vi "Adv_GetControlCurrentCapabilities_native.vi"(6 "LightField Setting":string, 8 "error in (no error)":errorcluster, 9 "Enum Class":refnum<k24>, 10 "Control":refnum<vi>, 11 "LightField Automation in":refnum<class "LightField Automation.lvclass">) -> (0 "error out":errorcluster, 3 "LightField Automation out":refnum<class "LightField Automation.lvclass">)   [LabVIEW 2015, in "LightField Automation.lvclass"]
uses:
  LightField Automation.lvclass
  C:/Program Files/Princeton Instruments/LightField/AddInViews/PrincetonInstruments.LightFieldViewV3.dll
  Program Files/Princeton Instruments/LightField/AddInViews/PrincetonInstruments.LightFieldViewV3.dll
  <vilib>/Utility/error.llb/DialogType.ctl
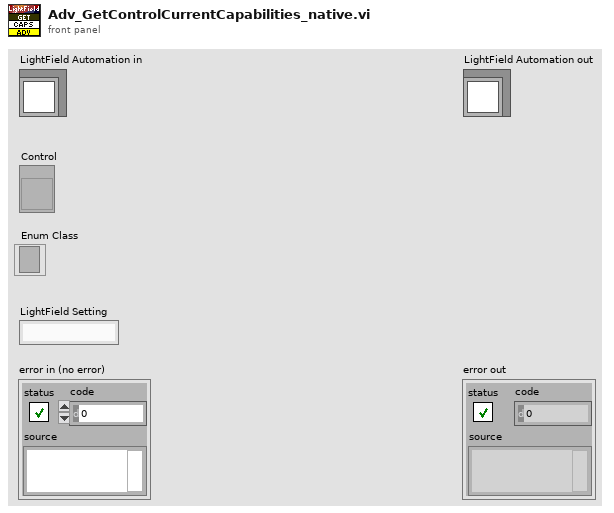
[diagram p1: front panel]
types:
  T1 = typedef "DialogType.ctl" = u16
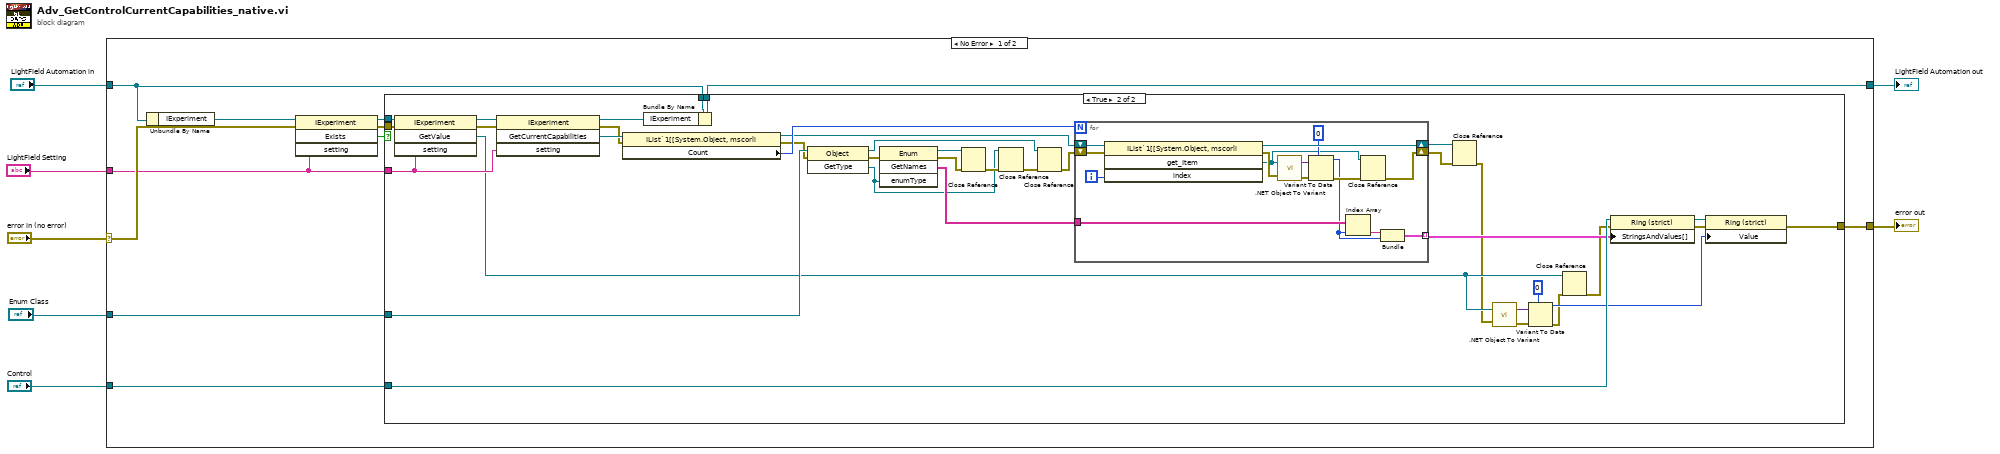
[diagram p0: block diagram]
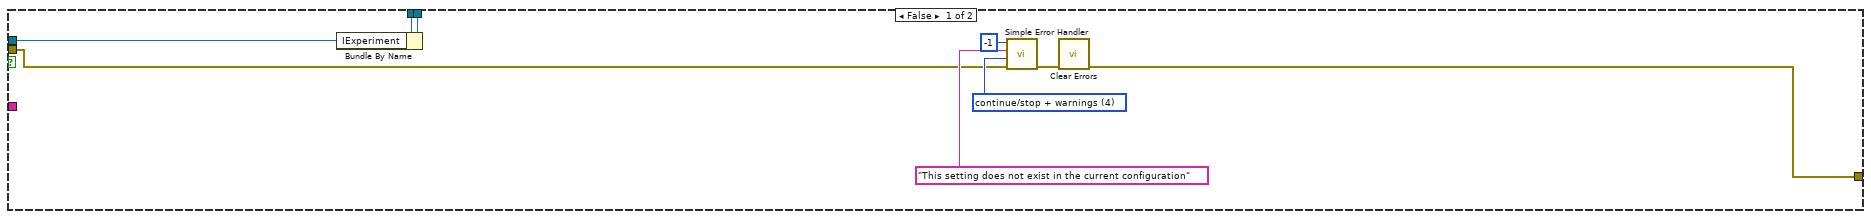
[diagram p2: hidden frame]
diagram:
  n1 = case shown="No Error" "error in (no error)" {
    selector: "error in (no error)" -> [w10 w82]
    tunnel: [w15 w82] -> w6
    tunnel: [w17 w81] -> w4
    tunnel: "LightField Automation in" -> [w18 w81]
    tunnel: "Control" -> [w16 _]
    tunnel: "LightField Setting" -> [w9 _]
    tunnel: "Enum Class" -> [w8 _]
    frame No Error {
      n2 = Unbundle By Name(w18) -> ("IExperiment"=w11:refnum<k24>)
      n3 = invoke class="IExperiment" method="Exists"(reference=w11, error in=w10, "setting"=w9) -> (reference out=w13:refnum<k24>, error out=w12:errorcluster, "Exists"=w14:bool)  [unwired: 1 in, 1 out]
      n4 = case shown="True" w14 {
        tunnel: w18 -> [w26 w65]
        tunnel: [w25 w64] -> w17
        tunnel: w16 -> [_ w60]
        tunnel: w13 -> [w27 w56]
        tunnel: w12 -> [w20 w53]
        tunnel: w9 -> [_ w49]
        tunnel: [w19 w43] -> w15
        tunnel: w8 -> [_ w42]
        frame False {
          w21 = T1 4 items=["no dialog", "OK message", "continue or stop message", "OK message + warnings", "continue/stop + warnings"] ("type of dialog (OK msg:1)")
          n5 = Bundle By Name(cluster=w26, "IExperiment"=w27) -> (w25:refnum<class "LightField Automation.lvclass">)
          n6 = call <vilib>:"Simple Error Handler.vi"("error code (no error:0)"=-1, "error source (\" \")"="This setting does not exist in the current configuration" ("source"), "type of dialog (OK msg:1)"=w21, "error in (no error)"=w20) -> ("error out"=w22:errorcluster)  [unwired: 1 in, 4 out]
          n7 = call <vilib>:"Clear Errors.vi"("error in (no error)"=w22) -> ("error out"=w19:errorcluster)  [unwired: 5 in, 1 out]
        }
        frame True {
          n8 = invoke class="IExperiment" method="GetValue"(reference=w56, error in=w53, "setting"=w49) -> (reference out=w55:refnum<k24>, error out=w54:errorcluster, "GetValue"=w39:refnum<k24>)  [unwired: 1 in, 1 out]
          n9 = invoke class="IExperiment" method="GetCurrentCapabilities"(reference=w55, error in=w54, "setting"=w49) -> (reference out=w59:refnum<k24>, error out=w57:errorcluster, "GetCurrentCapabilities"=w58:refnum<k24>)  [unwired: 1 in, 1 out]
          n10 = property class="IList`1[[System.Object, mscorli"(reference=w58, error in=w57) -> (reference out=w41:refnum<k24>, error out=w40:errorcluster, "Count"=w63:i32)
          n11 = Bundle By Name(cluster=w65, "IExperiment"=w59) -> (w64:refnum<class "LightField Automation.lvclass">)
          n12 = invoke class="Object" method="GetType"(reference=w42, error in=w40) -> (reference out=w34:refnum<k24>, error out=w38:errorcluster, "GetType"=w28:refnum<k24>)  [unwired: 1 in]
          n13 = invoke class="Enum" method="GetNames"(error in=w38, "enumType"=w28) -> (reference out=w36:refnum<k24>, error out=w31:errorcluster, "GetNames"=w37:string[])  [unwired: 2 in, 1 out]
          n14 = Close Reference(reference=w36, error in (no error)=w31) -> (error out=w29:errorcluster)
          n15 = Close Reference(reference=w28, error in (no error)=w29) -> (error out=w30:errorcluster)
          n16 = Close Reference(reference=w34, error in (no error)=w30) -> (error out=w35:errorcluster)
          n17 = for {
            N: w63 -> [_]
            shift-right: [w77] -> w61
            shift-left: w41 -> [w80]
            shift-right: [w71] -> w62
            shift-left: w35 -> [w79]
            tunnel: w37 -> [w69]
            tunnel: [w66] -> w44 mode=indexing
            i -> [w78]
            n18 = invoke class="IList`1[[System.Object, mscorli" method="get_Item"(reference=w80, error in=w79, "index"=w78) -> (reference out=w77:refnum<k24>, error out=w74:errorcluster, "get_Item"=w70:refnum<k24>)  [unwired: 1 in, 1 out]
            n19 = call <vilib>:".NET Object To Variant.vi"("error in (no error)"=w74, ".NET object"=w70) -> ("error out"=w76:errorcluster, "variant"=w75:variant)
            n20 = Variant To Data(error in=w76, type=0, Variant=w75) -> (data=w67:i32, error out=w72:errorcluster)
            n21 = Index Array(array=w69, index=w67) -> (element=w68:string)
            n22 = Close Reference(reference=w70, error in (no error)=w72) -> (error out=w71:errorcluster)
            n23 = Bundle(w68, w67) -> (w66:cluster{string, i32})  [unwired: 1 in]
          }
          n24 = Close Reference(reference=w61, error in (no error)=w62) -> (error out=w33:errorcluster)
          n25 = call <vilib>:".NET Object To Variant.vi"("error in (no error)"=w33, ".NET object"=w39) -> ("error out"=w52:errorcluster, "variant"=w51:variant)
          n26 = Variant To Data(error in=w52, type=0, Variant=w51) -> (data=w46:i32, error out=w45:errorcluster)
          n27 = Close Reference(reference=w39, error in (no error)=w45) -> (error out=w32:errorcluster)
          n28 = property class="Ring (strict)"(reference=w60, error in=w32, "StringsAndValues[]"=w44) -> (reference out=w48:refnum<vi>, error out=w47:errorcluster)
          n29 = property class="Ring (strict)"(reference=w48, error in=w47, "Value"=w46) -> (error out=w43:errorcluster)  [unwired: 1 out]
        }
      }
    }
    frame Error {
    }
  }
  "error out" <- w6
  "LightField Automation out" <- w4
